vi "Buffer Redraw Async.vi"(10 "Period s":dbl, 11 "LocalGraphBuffer in":refnum<class "LocalGraphBuffer.lvclass">) -> ()   [LabVIEW 2020, in "VolatusGUIElements.lvlib" / "LocalGraphBuffer.lvclass"]
uses:
  LocalGraphBuffer.lvclass
  LocalGraphBuffer.lvclass/LocalGraphBuffer.ctl
  Decimation Params.ctl
  VolatusGUIElements.lvlib
panel:
  out "XY Graph 2":cluster{dbl[], dbl[]}[](graph)
  out "XY Graph":cluster{"elements":dbl[], "elements":dbl[]}[](graph)
  out "Data":dbl[](array[numeric])
  out "Timestamp":dbl format="%<%H:%M:%S%3u>T"
  out "Channels":string[](array[string])
  out "i":i32
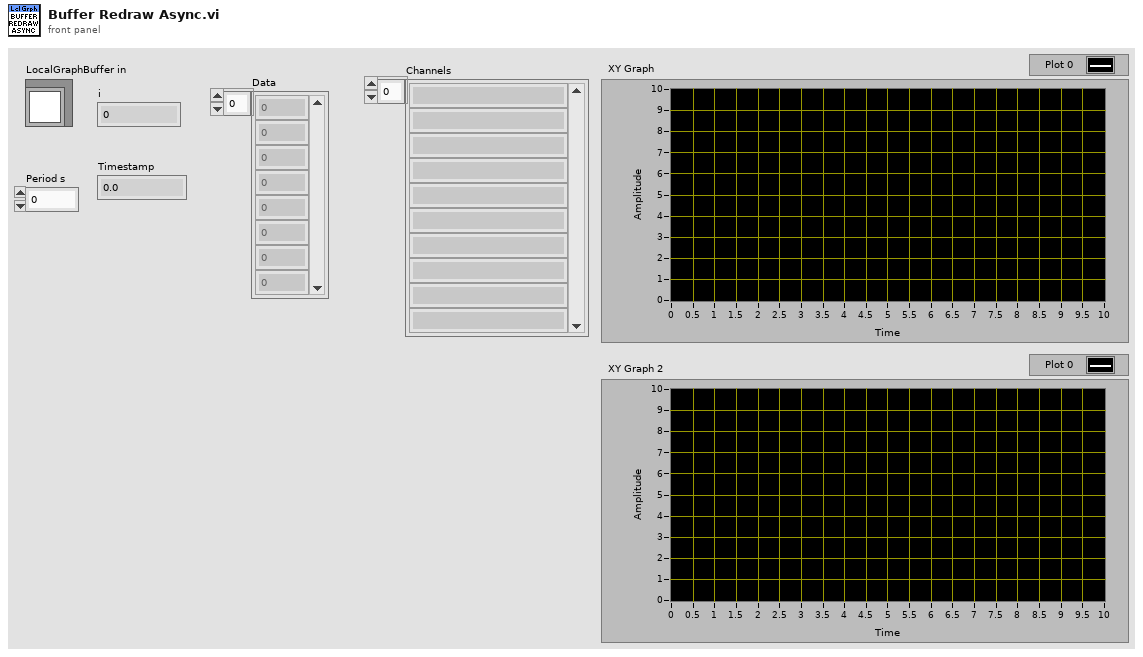
[diagram p1: front panel]
types:
  T1 = typedef "VolatusGUIElements.lvlib/LocalGraphBuffer.lvclass/Plot.ctl" = cluster{"Data Q":refnum<queue>, "Time Q":refnum<queue>, "Group":string, "Channel Index":i32}
  T2 = typedef "VolatusGUIElements.lvlib/LocalGraphBuffer.lvclass/Group Sub.ctl" = cluster{"Plot Indices":i32[]}
  T3 = typedef "VolatusGUIElements.lvlib/Decimation Params.ctl" = cluster{"Width":i32, "Start":dbl, "End":dbl}
  T4 = typedef "Vecto.lvlib/Subscribed Data.ctl" = cluster{"Group":string, "Timestamp":dbl, "Data":dbl[]}
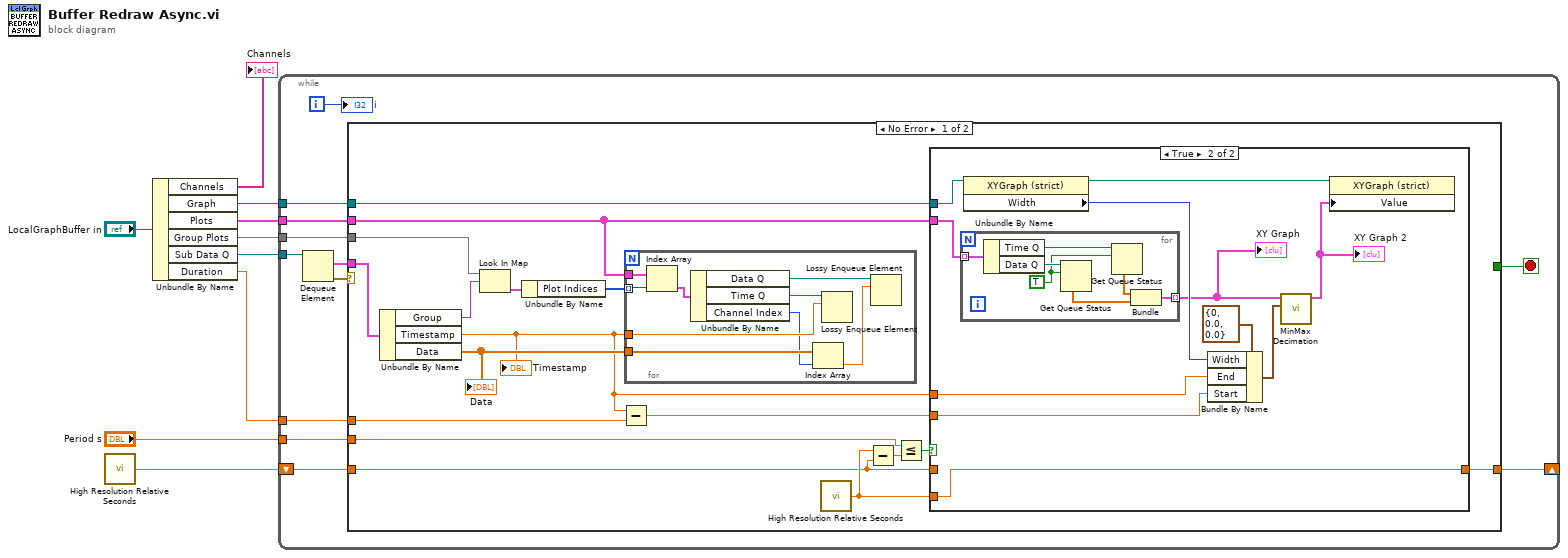
[diagram p0: block diagram]
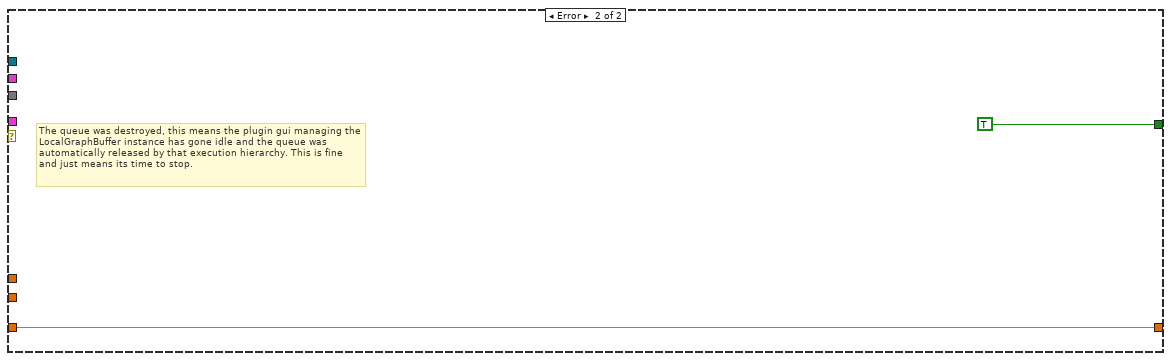
[diagram p3: hidden frame]
diagram:
  n1 = call <vilib>:"High Resolution Relative Seconds.vi"() -> ("relative seconds"=w8:dbl)
  n2 = Unbundle By Name("LocalGraphBuffer in") -> ("Channels"=→"Channels":string[], "Graph"=w7:refnum<vi>, "Plots"=w6:T1[], "Group Plots"=w3:map{string, T2}, "Sub Data Q"=w4:refnum<queue>, "Duration"=w1:dbl)
  n3 = while {
    tunnel: "Period s" -> [w21]
    shift-right: [w19] -> _
    shift-left: w8 -> [w20]
    tunnel: w7 -> [w18]
    tunnel: w6 -> [w15]
    tunnel: w4 -> [w17]
    tunnel: w3 -> [w16]
    tunnel: w1 -> [w10]
    i -> [w11]
    stop <- w12 stop-if-true
    n4 = Dequeue Element(queue=w17) -> (element=w14:T4, error out=w13:errorcluster)  [unwired: 2 in, 2 out]
    n5 = case shown="No Error" w13 {
      tunnel: w21 -> [w37 _]
      tunnel: w20 -> [w34 w68]
      tunnel: [w33 w68] -> w19
      tunnel: w18 -> [w32 _]
      tunnel: w16 -> [w29 _]
      tunnel: w15 -> [w28 _]
      tunnel: w14 -> [w27 _]
      tunnel: [_ TRUE] -> w12
      tunnel: w10 -> [w24 _]
      frame No Error {
        n6 = Unbundle By Name(w27) -> ("Group"=w25:string, "Timestamp"=w22:dbl, "Data"=w26:dbl[])
        "Timestamp" <- w22
        "Data" <- w26
        n7 = Look In Map(map=w29, key=w25) -> (value=w31:T2)  [unwired: 1 in, 1 out]
        n8 = Unbundle By Name(w31) -> ("Plot Indices"=w30:i32[])
        n9 = Subtract(x=w22, y=w24) -> (x-y=w23:dbl)
        n10 = for {
          tunnel: w22 -> [w43]
          tunnel: w30 -> [w40] mode=indexing
          tunnel: w28 -> [w46]
          tunnel: w26 -> [w47]
          n11 = Index Array(array=w46, index=w40) -> (element=w45:T1)
          n12 = Unbundle By Name(w45) -> ("Data Q"=w42:refnum<queue>, "Time Q"=w44:refnum<queue>, "Channel Index"=w39:i32)
          n13 = Index Array(array=w47, index=w39) -> (element=w41:dbl)
          n14 = Lossy Enqueue Element(queue=w44, element=w43) -> ()  [unwired: 1 in, 4 out]
          n15 = Lossy Enqueue Element(queue=w42, element=w41) -> ()  [unwired: 1 in, 4 out]
        }
        n16 = call <vilib>:"High Resolution Relative Seconds.vi"() -> ("relative seconds"=w35:dbl)
        n17 = Subtract(x=w35, y=w34) -> (x-y=w38:dbl)
        n18 = Less Or Equal?(x=w37, y=w38) -> (x <= y?=w36:bool)
        n19 = case shown="True" w36 {
          tunnel: w35 -> [_ w58]
          tunnel: w34 -> [w48 _]
          tunnel: [w48 w58] -> w33
          tunnel: w32 -> [_ w57]
          tunnel: w28 -> [_ w56]
          tunnel: w23 -> [_ w52]
          tunnel: w22 -> [_ w51]
          frame False {
          }
          frame True {
            n20 = for {
              tunnel: w56 -> [w66] mode=indexing
              tunnel: [w60] -> w50 mode=indexing
              w63 = TRUE ("return elements? (F)")
              n21 = Unbundle By Name(w66) -> ("Time Q"=w64:refnum<queue>, "Data Q"=w65:refnum<queue>)
              n22 = Get Queue Status(queue=w65, return elements? (F)=w63) -> (elements=w61:dbl[])  [unwired: 1 in, 7 out]
              n23 = Get Queue Status(queue=w64, return elements? (F)=w63) -> (elements=w62:dbl[])  [unwired: 1 in, 7 out]
              n24 = Bundle("elements"=w62, "elements"=w61) -> (w60:cluster{"elements":dbl[], "elements":dbl[]})  [unwired: 1 in]
            }
            "XY Graph" <- w50
            n25 = property class="XYGraph (strict)"(reference=w57) -> (reference out=w59:refnum<vi>, "Width"=w55:u32)  [unwired: 1 in, 1 out]
            n26 = Bundle By Name(cluster=T3 {"Width"=0, "Start"=0.0, "End"=0.0} ("Params"), "Width"=w55, "End"=w51, "Start"=w52) -> (w53:T3)
            n27 = call "MinMax Decimation.vi"("Params"=w53, "XY Data"=w50) -> ("MinMax Data"=w49:cluster{dbl[], dbl[]}[])  [unwired: 9 in]
            "XY Graph 2" <- w49
            n28 = property class="XYGraph (strict)"(reference=w59, "Value"=w49) -> ()  [unwired: 1 in, 2 out]
          }
        }
      }
      frame Error {
        # "The queue was destroyed, this means the plugin gui managing the LocalGraphBuffer instance has gone idle and the queue was automatically released by that execution hierarchy. This is fine and just means its time to stop."
      }
    }
    "i" <- w11
  }
